vi "flow_queue_end.vi"(8 "error in (no error)":errorcluster caption="エラー入力（エラーなし）", 11 "flow_refnum":refnum<queue>[](array[refnum])) -> (0 "error out":errorcluster caption="エラー出力")   [LabVIEW 2017]
uses:
  flow_queue_datatype.ctl
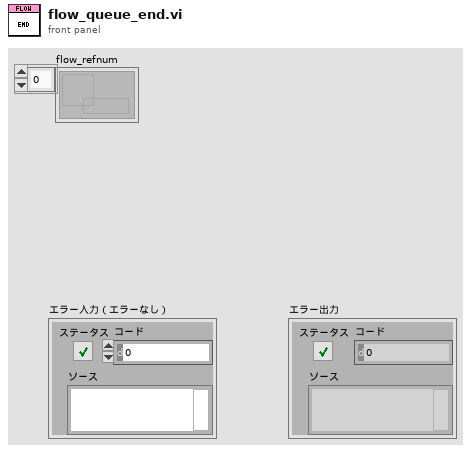
[diagram p1: front panel]
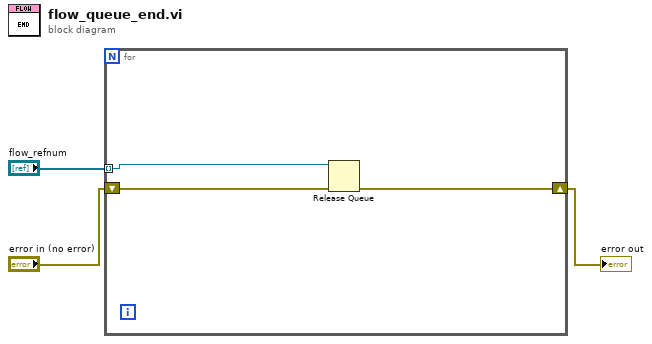
[diagram p0: block diagram]
diagram:
  n1 = for {
    tunnel: "flow_refnum" -> [w6] mode=indexing
    shift-right: [w4] -> w2
    shift-left: "error in (no error)" -> [w5]
    n2 = Release Queue(queue=w6, error in (no error)=w5) -> (error out=w4:errorcluster)  [unwired: 1 in, 2 out]
  }
  "error out" <- w2
